vi "LJM logger shift scaling equations.vi"(4 "Error In (no error)":errorcluster, 5 "Scaling Equations In":string[](array[string])=["y=a", "y=b", "y=c", "y=d", "y=e", "y=f", "y=g", "y=h", "y=i", "y=j", "y=k", "y=l", "y=m", "y=n", "y=o", "y=p", "y=a2", "y=b2", "y=c2", "y=d2", "y=e2", "y=f2", "y=g2", "y=h2", "y=i2", "y=j2", "y=k2", "y=l2", "y=m2", "y=n2", "y=o2", "y=p2", "y=a3", "y=b3", "y=c3", "y=d3", "y=e3", "y=f3", "y=g3", "y=h3", "y=i3", "y=j3", "y=k3", "y=l3", "y=m3", "y=n3", "y=o3", "y=p3", "y=a4", "y=b4", "y=c4", "y=d4", "y=e4", "y=f4", "y=g4", "y=h4", "y=i4", "y=j4", "y=k4", "y=l4", "y=m4", "y=n4", "y=o4", "y=p4", "y=a5", "y=b5", "y=c5", "y=d5", "y=e5", "y=f5", "y=g5", "y=h5", "y=i5", "y=j5", "y=k5", "y=l5", "y=m5", "y=n5", "y=o5", "y=p5", "y=a6", "y=b6", "y=c6", "y=d6", "y=e6", "y=f6", "y=g6", "y=h6", "y=i6", "y=j6", "y=k6", "y=l6", "y=m6", "y=n6", "y=o6", "y=p6", "y=a7", "y=b7", "y=c7", "y=d7"], 6 "Index Shift Value":i32=-1, 7 "Modification Index":i32=2) -> (0 "Error Out":errorcluster, 1 "Scaling Equations Out":string[](array[string]))   [LabVIEW 2026]
panel:
  # "This VI will shift scaling equation variables up or down so you can easily insert or delete rows in the logger. Note that this VI does not actually delete or insert any elements."
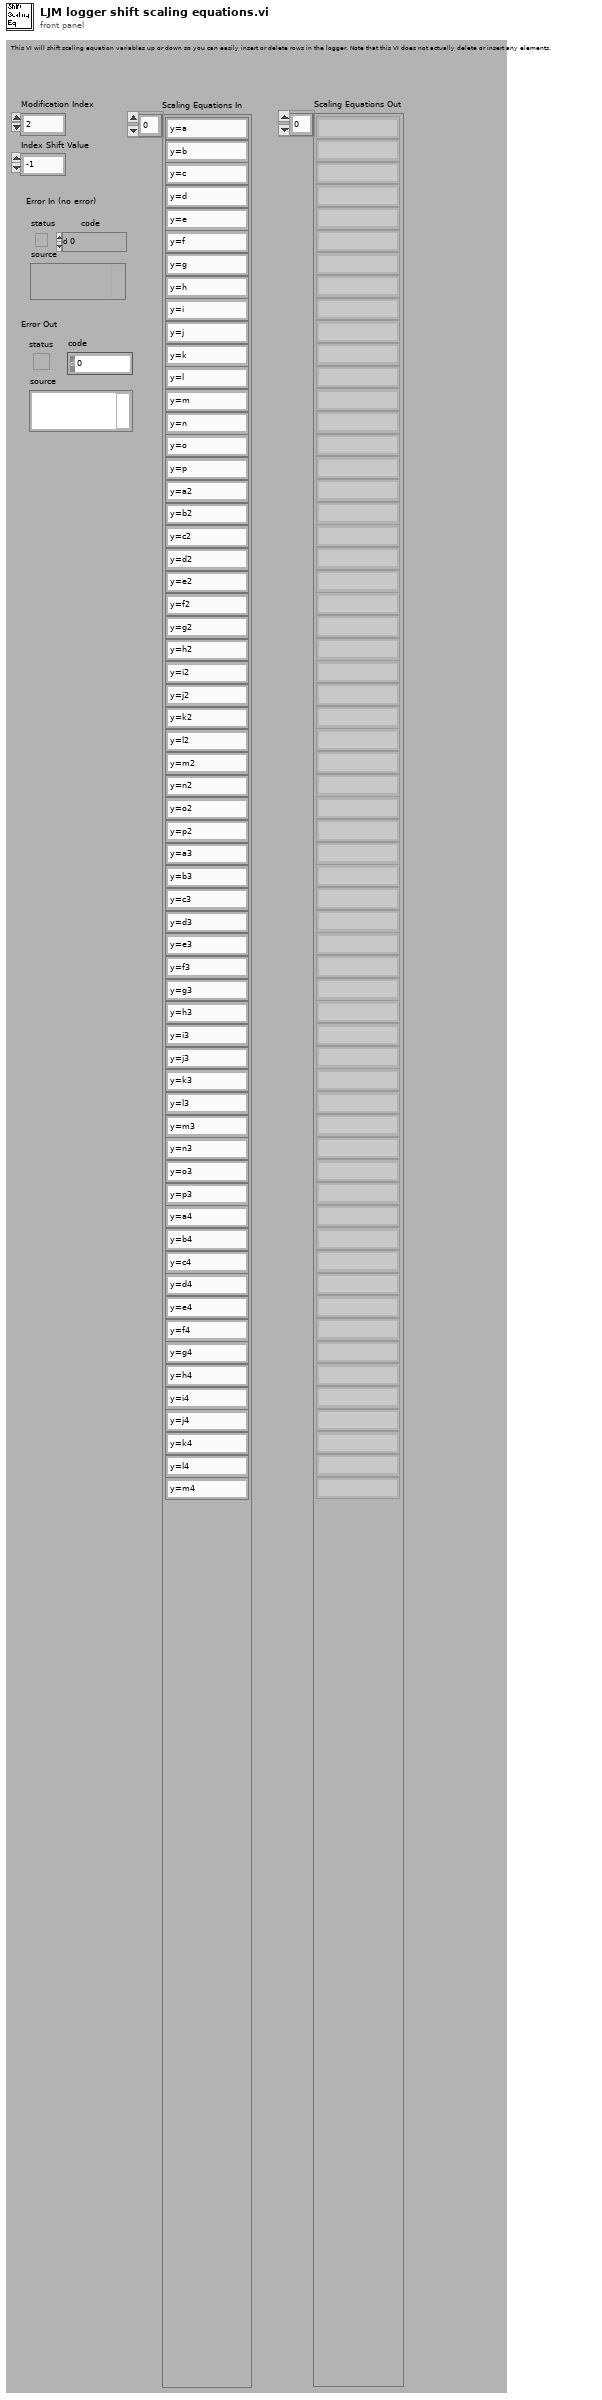
[diagram p1: front panel]
types:
  T1 = typedef "Program Config Cluster.ctl" = cluster{"Data File Prefix":string, "Scan Rate (Hz)":dbl, "Graph History":i32, "# Channels":i32, "Disable Scaling":bool, "Max File Size (Bytes)":i32, "Channel Setup":T2, "Interval (ms)":u32, "Write To File":bool, "Log Every n Scans":i32}
  T2 = typedef "Channel Setup.ctl" = cluster{"Name":string[], string, "Scaling Equation":string[], string, "Graph?":bool[]}
  T3 = cluster{"regular expression":string, "regular expression":string}
  T4 = cluster{"regular expression":string, "regular expression":string}[]
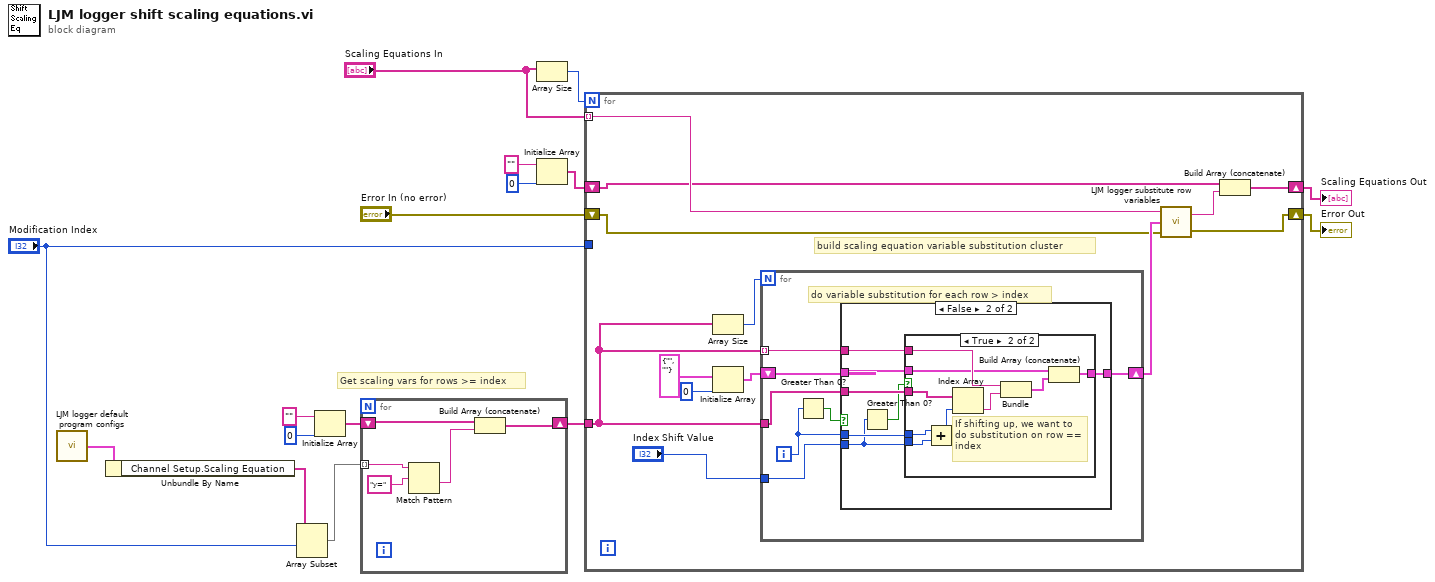
[diagram p0: block diagram]
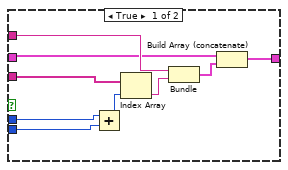
[diagram p2: hidden frame]
diagram:
  # "Get scaling vars for rows >= index"
  n1 = call "LJM logger default program configs.vi"() -> ("Program Configs"=w15:T1)  [unwired: 1 in]
  n2 = Unbundle By Name(w15) -> ("Channel Setup.Scaling Equation"=w14:string[])
  n3 = Array Subset(array=w14, index="Modification Index") -> (w13:string[])  [unwired: 1 in]
  n4 = Initialize Array("" ("regular expression"), 0 ("dimension size")) -> (w10:string[])
  n5 = for {
    tunnel: w13 -> [w20] mode=indexing
    shift-right: [w17] -> w9
    shift-left: w10 -> [w19]
    n6 = Match Pattern(string=w20, regular expression="y=") -> (after substring=w18:string)  [unwired: 1 in, 3 out]
    n7 = Build Array (concatenate)(w19, w18) -> (w17:string[])
  }
  n8 = Array Size(array="Scaling Equations In") -> (size(s)=w16:i32)
  n9 = Initialize Array("" ("regular expression"), 0 ("dimension size")) -> (w6:string[])
  n10 = for {
    N: w16 -> [_]
    tunnel: "Modification Index" -> [_]
    tunnel: "Scaling Equations In" -> [w34] mode=indexing
    tunnel: w9 -> [w33]
    shift-right: [w26] -> w5
    shift-left: w6 -> [w25]
    shift-right: [w22] -> w1
    shift-left: "Error In (no error)" -> [w23]
    # "build scaling equation variable substitution cluster"
    n11 = Array Size(array=w33) -> (size(s)=w32:i32)
    n12 = Initialize Array(T3 {"regular expression"="", "regular expression"=""}, 0 ("dimension size")) -> (w29:T4)
    n13 = for {
      N: w32 -> [_]
      tunnel: w33 -> [w41] mode=indexing
      tunnel: w33 -> [w40]
      shift-right: [w39] -> w28
      shift-left: w29 -> [w36]
      tunnel: "Index Shift Value" -> [w35]
      i -> [w37]
      # "do variable substitution for each row > index"
      n14 = Greater Than 0?(x=w37) -> (x > 0?=w38:bool)
      n15 = case shown="False" w38 {
        tunnel: w41 -> [w50 w57]
        tunnel: w40 -> [w49 w56]
        tunnel: w37 -> [w43 w53]
        tunnel: [w45 w54] -> w39
        tunnel: w36 -> [w47 w55]
        tunnel: w35 -> [w42 w52]
        frame True {
          n16 = Add(x=w43, y=w42) -> (x+y=w44:i32)
          n17 = Index Array(array=w49, index=w44) -> (element=w48:string)
          n18 = Bundle("regular expression"=w50, "regular expression"=w48) -> (w46:T3)  [unwired: 1 in]
          n19 = Build Array (concatenate)(w47, w46) -> (w45:T4)
        }
        frame False {
          n20 = Greater Than 0?(x=w52) -> (x > 0?=w51:bool)
          n21 = case shown="True" w51 {
            tunnel: w57 -> [_ w67]
            tunnel: w56 -> [_ w66]
            tunnel: w55 -> [w58 w64]
            tunnel: [w58 w62] -> w54
            tunnel: w53 -> [_ w60]
            tunnel: w52 -> [_ w59]
            frame False {
            }
            frame True {
              # "If shifting up, we want to do substitution on row == index"
              n22 = Add(x=w60, y=w59) -> (x+y=w61:i32)
              n23 = Index Array(array=w66, index=w61) -> (element=w65:string)
              n24 = Bundle("regular expression"=w67, "regular expression"=w65) -> (w63:T3)  [unwired: 1 in]
              n25 = Build Array (concatenate)(w64, w63) -> (w62:T4)
            }
          }
        }
      }
    }
    n26 = call "LJM logger substitute row variables.vi"("error in (no error)"=w23, "Substitution Rules"=w28, "original formula"=w34) -> ("error out"=w22:errorcluster, "formula after substitution"=w27:string)
    n27 = Build Array (concatenate)(w25, w27) -> (w26:string[])
  }
  "Scaling Equations Out" <- w5
  "Error Out" <- w1
